vi "svl_Limit x and y Axes.vi"(2 "y scale":cluster{"y min":dbl, "y max":dbl} {"y max" format="%.2f"; "y min" format="%.2f"}, 3 "x scale":cluster{"x min":dbl, "x max":dbl} {"x max" format="%.2f"; "x min" format="%.2f"}, 4 "scale info":cluster{"x scale":dbl[], "y scale":dbl[]} {"y scale" format="%.2f"; "x scale" format="%.2f"}) -> (0 "subset info":T1, 1 "scale subset":cluster{"x scale":dbl[], "y scale":dbl[]} {"y scale" format="%.2f"; "x scale" format="%.2f"})   [LabVIEW 2017]
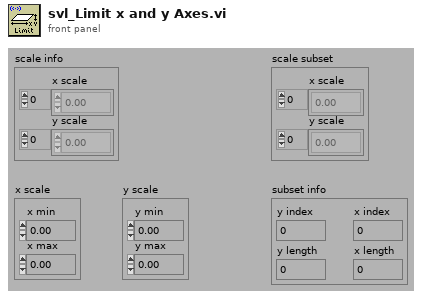
[diagram p1: front panel]
types:
  T1 = cluster{"y index":i32, "y length":i32, "x index":i32, "x length":i32}
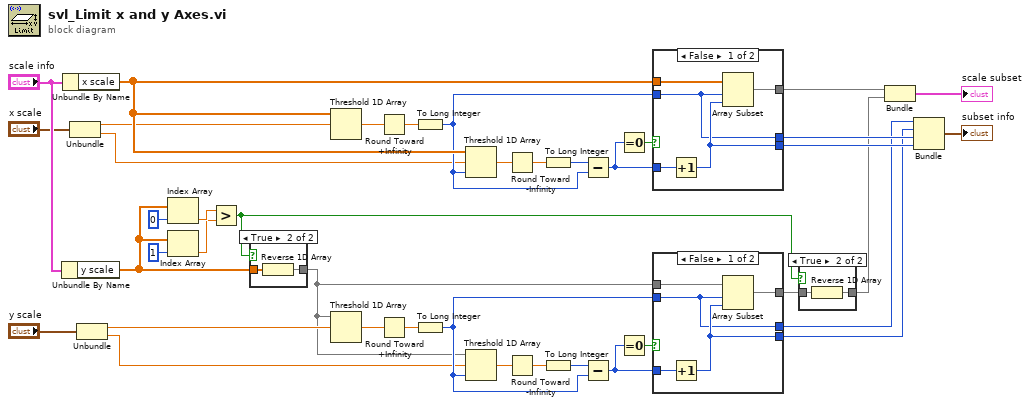
[diagram p0: block diagram]
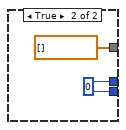
[diagram p4: hidden frame]
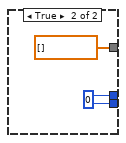
[diagram p5: hidden frame]
diagram:
  n1 = Unbundle By Name("scale info") -> ("y scale"=w5:dbl[])
  n2 = Unbundle By Name("scale info") -> ("x scale"=w38:dbl[])
  n3 = Unbundle("x scale") -> ("x min"=w20:dbl, "x max"=w18:dbl)
  n4 = Unbundle("y scale") -> ("y min"=w17:dbl, "y max"=w15:dbl)
  n5 = Index Array(array=w5, index=0) -> (element=w7:dbl)
  n6 = Index Array(array=w5, index=1) -> (element=w6:dbl)
  n7 = Greater?(x=w7, y=w6) -> (0:w1:bool)
  n8 = case shown="True" w1 {
    tunnel: w5 -> [w41 w43]
    tunnel: [w41 w42] -> w4
    frame False {
    }
    frame True {
      n9 = Reverse 1D Array(array=w43) -> (reversed array=w42:dbl[])
    }
  }
  n10 = Threshold 1D Array(2:w20, 3:w38) -> (0:w40:dbl)  [unwired: 1 in]
  n11 = Threshold 1D Array(2:w17, 3:w4) -> (0:w24:dbl)  [unwired: 1 in]
  n12 = Round Toward +Infinity(x=w40) -> (ceil(x): smallest int >= x=w39:dbl)
  n13 = Round Toward +Infinity(x=w24) -> (ceil(x): smallest int >= x=w25:dbl)
  n14 = To Long Integer(number=w39) -> (32bit integer=w34:i32)
  n15 = To Long Integer(number=w25) -> (32bit integer=w29:i32)
  n16 = Threshold 1D Array(1:w34, 2:w18, 3:w38) -> (0:w37:dbl)
  n17 = Threshold 1D Array(1:w29, 2:w15, 3:w4) -> (0:w26:dbl)
  n18 = Round Toward -Infinity(1:w37) -> (0:w36:dbl)
  n19 = Round Toward -Infinity(1:w26) -> (0:w27:dbl)
  n20 = To Long Integer(number=w36) -> (32bit integer=w35:i32)
  n21 = To Long Integer(number=w27) -> (32bit integer=w28:i32)
  n22 = Subtract(x=w35, y=w34) -> (x-y=w33:i32)
  n23 = Subtract(x=w28, y=w29) -> (x-y=w30:i32)
  n24 = Equal To 0?(x=w33) -> (x = 0?=w32:bool)
  n25 = Equal To 0?(x=w30) -> (x = 0?=w31:bool)
  n26 = case shown="False" w32 {
    tunnel: w38 -> [w48 _]
    tunnel: w34 -> [w44 _]
    tunnel: w33 -> [w47 _]
    tunnel: [w46 dbl[] []] -> w22
    tunnel: [w45 w49] -> w13
    tunnel: [w44 w49] -> w12
    frame False {
      n27 = Increment(x=w47) -> (x+1=w45:i32)
      n28 = Array Subset(array=w48, index=w44, length=w45) -> (w46:dbl[])
    }
    frame True {
      w49 = 0
    }
  }
  n29 = case shown="False" w31 {
    tunnel: w4 -> [w55 _]
    tunnel: w29 -> [w51 _]
    tunnel: w30 -> [w54 _]
    tunnel: [w53 dbl[] []] -> w3
    tunnel: [w52 w56] -> w10
    tunnel: [w51 w56] -> w11
    frame False {
      n30 = Increment(x=w54) -> (x+1=w52:i32)
      n31 = Array Subset(array=w55, index=w51, length=w52) -> (w53:dbl[])
    }
    frame True {
      w56 = 0
    }
  }
  n32 = case shown="True" w1 {
    tunnel: w3 -> [w58 w60]
    tunnel: [w58 w59] -> w2
    frame False {
    }
    frame True {
      n33 = Reverse 1D Array(array=w60) -> (reversed array=w59:dbl[])
    }
  }
  n34 = Bundle(w22, w2) -> (→"scale subset":cluster{dbl[], dbl[]})  [unwired: 1 in]
  n35 = Bundle(w11, w10, w12, w13) -> (→"subset info":cluster{i32, i32, i32, i32})  [unwired: 1 in]
